vi "Get Mapped Memory Information.vi"(1 "Mapped Memory Access Image Greyscale in":refnum<class "Mapped Memory Access Image Greyscale.lvclass">) -> (0 "Raw Memory Information":T1)   [LabVIEW 2020, in "g_ar_toolkit.image.lvlib" / "Mapped Memory Access Image Greyscale.lvclass"]
uses:
  Mapped Memory Access Image Greyscale.lvclass
  Raw Memory Information.ctl
  Raw Memory Information Dimension.ctl
  Mapped Memory Access Image Greyscale.lvclass/Mapped Memory Access Image Greyscale.ctl
  g_ar_toolkit.image.lvlib
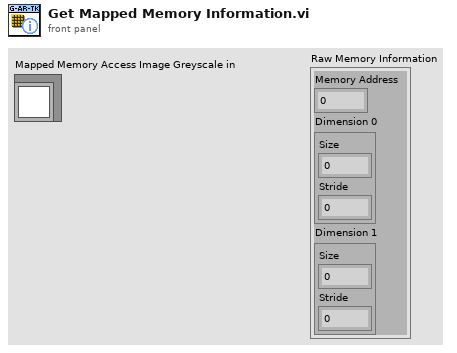
[diagram p1: front panel]
types:
  T1 = typedef "g_ar_toolkit.image.lvlib/Raw Memory Information.ctl" = cluster{"Memory Address":u64, "Dimension 0":T2, "Dimension 1":T2}
  T2 = typedef "g_ar_toolkit.image.lvlib/Raw Memory Information Dimension.ctl" = cluster{"Size":u16, "Stride":u32}
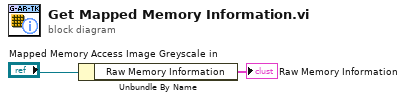
[diagram p0: block diagram]
diagram:
  n1 = Unbundle By Name("Mapped Memory Access Image Greyscale in") -> ("Raw Memory Information"=→"Raw Memory Information":T1)
